vi "CDMA_RxMsgDecode.vi"(8 "error in (no error)":errorcluster caption="错误输入（无错误）", 10 "ch_decode_data":dbl[](array[numeric]), 11 "Path In":path) -> (0 "error out":errorcluster caption="错误输出", 2 "char_msg":string, 3 "Path  Out":path)   [LabVIEW 2015]
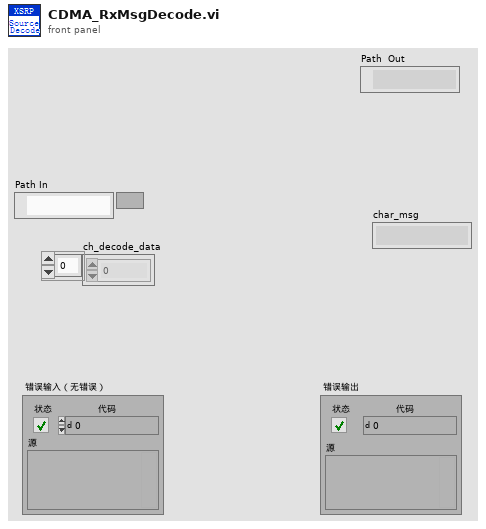
[diagram p1: front panel]
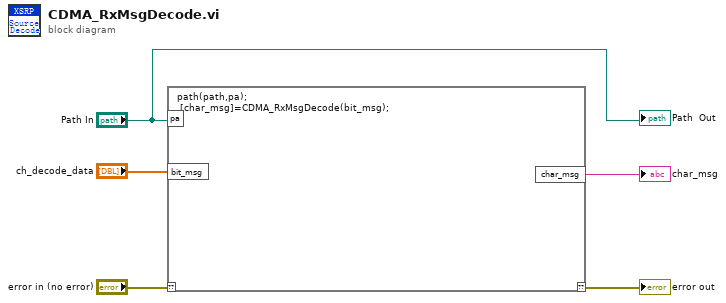
[diagram p0: block diagram]
diagram:
  n1 = script code="path(path,pa);\n [char_msg]=CDMA_RxMsgDecode(bit_msg);"("??"="error in (no error)", "pa"="Path In", "bit_msg"="ch_decode_data") -> ("??"=→"error out":errorcluster, "char_msg"=→"char_msg":string)
  "Path  Out" <- "Path In"
